vi "FTW-Request-Core-InterpretResponse.vi"(0 "Raw Response":T1, 5 "Expected Request Header":string, 11 "error in":errorcluster) -> (4 "InterpretedResponse":T1, 15 "error out":errorcluster)   [LabVIEW 2015]
doc: "Sends a response message back to the requesting client. This message is attempts to send unconditionally of incoming error. Take caution to wire a sanitized error into this function, because it will be repeated back onto the client. Said another way, an error generated while processing the request will be not only thrown on the request handler, but also on the client as well."
uses:
  core/type/FTW-Type-JSON.ctl
  error/FTW-ERR-ExceptionType.ctl
panel:
  # "Inputs"
  # "Outputs"
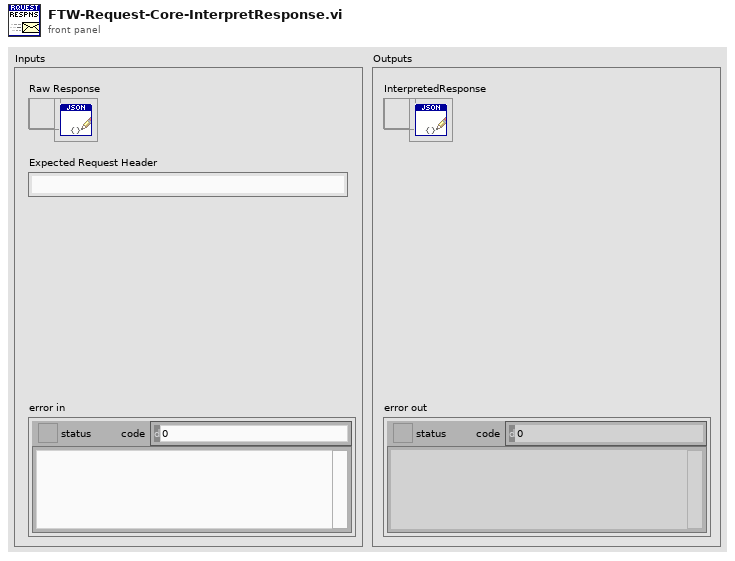
[diagram p1: front panel]
types:
  T1 = typedef "FTW-Type-JSON.ctl" = refnum<data-value>
  T2 = typedef "FTW-JSON-Type.ctl" = enum8{"Not Found", "Object", "Array", "String", "Number", "Boolean", "null"}
  T3 = typedef "FTW-ERR-ExceptionType.ctl" = enum16{"OK", "Info", "Warning", "Error"}
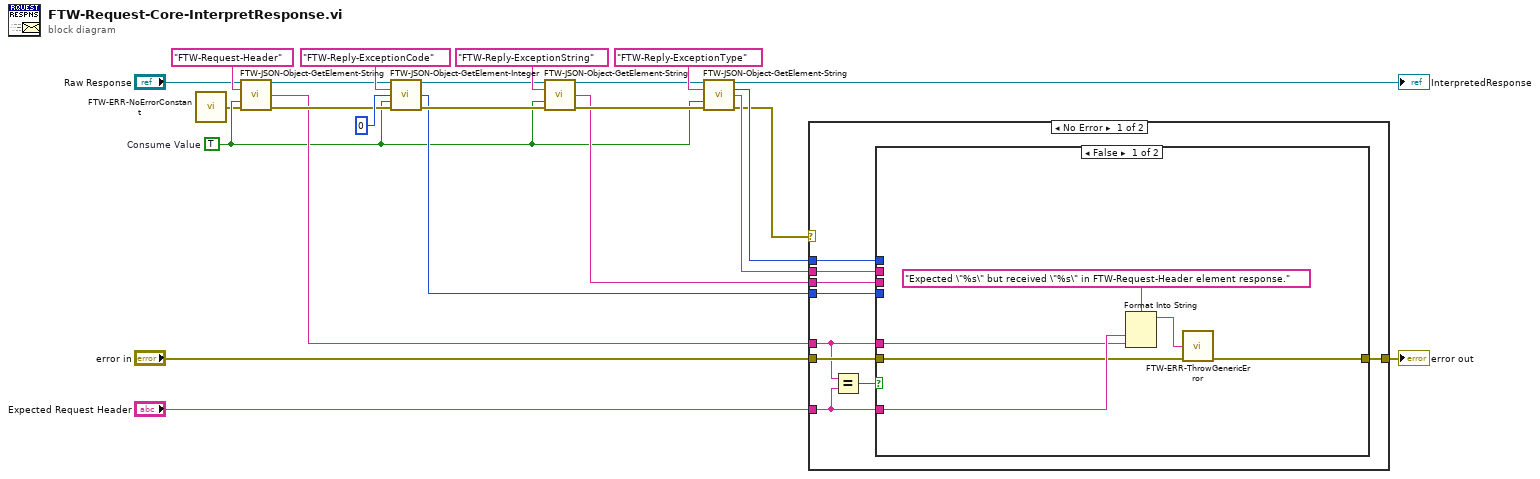
[diagram p0: block diagram]
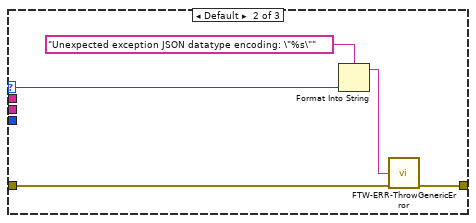
[diagram p3: hidden frame]
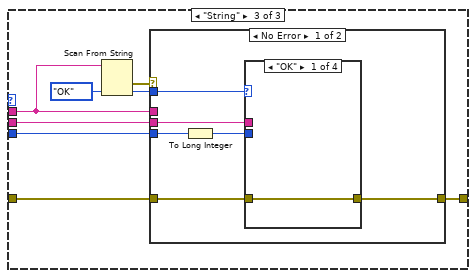
[diagram p4: hidden frame]
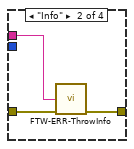
[diagram p5: hidden frame]
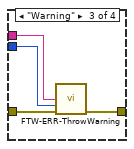
[diagram p6: hidden frame]
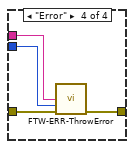
[diagram p7: hidden frame]
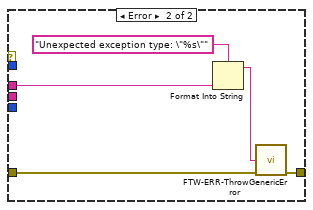
[diagram p8: hidden frame]
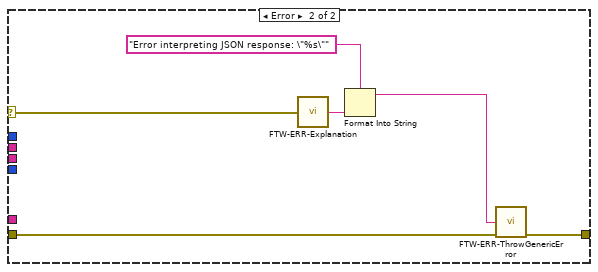
[diagram p9: hidden frame]
diagram:
  w5 = TRUE  # Consume Value
  n1 = call "FTW-ERR-NoErrorConstant.vi"() -> ("no error"=w3:errorcluster)
  n2 = call "FTW-JSON-Object-GetElement-String.vi"("JSON"="Raw Response", "Key"="FTW-Request-Header", "Consume Value"=w5, "error in"=w3) -> ("JSON out"=w8:T1, "Value"=w6:string, "error out"=w7:errorcluster)  [unwired: 8 in, 1 out]
  n3 = call "FTW-JSON-Object-GetElement-Integer.vi"("JSON"=w8, "Key"="FTW-Reply-ExceptionCode", "Default Value"=i64 0, "Consume Value"=w5, "error in"=w7) -> ("JSON out"=w18:T1, "Value"=w13:i64, "error out"=w17:errorcluster)  [unwired: 7 in, 1 out]
  n4 = call "FTW-JSON-Object-GetElement-String.vi"("JSON"=w18, "Key"="FTW-Reply-ExceptionString", "Consume Value"=w5, "error in"=w17) -> ("JSON out"=w15:T1, "Value"=w12:string, "error out"=w14:errorcluster)  [unwired: 8 in, 1 out]
  n5 = call "FTW-JSON-Object-GetElement-String.vi"("JSON"=w15, "Key"="FTW-Reply-ExceptionType", "Consume Value"=w5, "error in"=w14) -> ("JSON out"=→"InterpretedResponse":T1, "JSON Element Type"=w10:T2, "Value"=w11:string, "error out"=w2:errorcluster)  [unwired: 8 in]
  n6 = case shown="No Error" w2 {
    selector: w2 -> [_ w84]
    tunnel: [w30 w85] -> w23
    tunnel: "error in" -> [w31 w88]
    tunnel: w13 -> [w33 _]
    tunnel: w12 -> [w29 _]
    tunnel: w11 -> [w28 _]
    tunnel: w10 -> [w32 _]
    tunnel: w6 -> [w25 _]
    tunnel: "Expected Request Header" -> [w26 _]
    frame No Error {
      n7 = Equal?(x=w25, y=w26) -> (x = y?=w27:bool)
      n8 = case shown="False" w27 {
        tunnel: w33 -> [_ w45]
        tunnel: w32 -> [_ w44]
        tunnel: w31 -> [w35 w43]
        tunnel: [w34 w42] -> w30
        tunnel: w29 -> [_ w41]
        tunnel: w28 -> [_ w40]
        tunnel: w26 -> [w37 _]
        tunnel: w25 -> [w36 _]
        frame False {
          n9 = Format Into String(format string="Expected \"%s\" but received \"%s\" in FTW-Request-Header element response.", w37, w36) -> (resulting string=w39:string)  [unwired: 2 in, 1 out]
          n10 = call "FTW-ERR-ThrowGenericError.vi"("Error Message"=w39, "error in"=w35) -> ("error out"=w34:errorcluster)  [unwired: 13 in]
        }
        frame True {
          n11 = case shown="\"Not Found\", \"null\"" w44 {
            selector: w44 -> [_ w48 _]
            tunnel: w43 -> [w46 w51 w57]
            tunnel: [w46 w50 w56] -> w42
            tunnel: w40 -> [_ _ w55]
            tunnel: w41 -> [_ _ w53]
            tunnel: w45 -> [_ _ w52]
            frame "Not Found", "null" {
              # "No Exception"
            }
            frame Default {
              n12 = Format Into String(format string="Unexpected exception JSON datatype encoding: \"%s\"", w48) -> (resulting string=w47:string)  [unwired: 2 in, 1 out]
              n13 = call "FTW-ERR-ThrowGenericError.vi"("Error Message"=w47, "error in"=w51) -> ("error out"=w50:errorcluster)  [unwired: 13 in]
            }
            frame "String" {
              n14 = Scan From String(input string=w55, default 1=FTW-ERR-ExceptionType."OK" ("Exception")) -> (error out=w58:errorcluster, output 1=w54:T3)  [unwired: 3 in, 2 out]
              n15 = case shown="No Error" w58 {
                tunnel: w57 -> [w63 w82]
                tunnel: [w64 w81] -> w56
                tunnel: w55 -> [_ w78]
                tunnel: w54 -> [w65 _]
                tunnel: w52 -> [w61 _]
                tunnel: w53 -> [w62 _]
                frame No Error {
                  n16 = To Long Integer(number=w61) -> (32bit integer=w60:i32)
                  n17 = case shown="\"OK\"" w65 {
                    tunnel: [w66 w68 w72 w76] -> w64
                    tunnel: w63 -> [w66 w69 w73 w77]
                    tunnel: w62 -> [_ w67 w71 w75]
                    tunnel: w60 -> [_ _ w70 w74]
                    frame "OK" {
                    }
                    frame "Info" {
                      n18 = call "FTW-ERR-ThrowInfo.vi"("Informational Message"=w67, "error in"=w69) -> ("error out"=w68:errorcluster)  [unwired: 13 in]
                    }
                    frame "Warning" {
                      n19 = call "FTW-ERR-ThrowWarning.vi"("Warning Message"=w71, "Warning Code"=w70, "error in"=w73) -> ("error out"=w72:errorcluster)  [unwired: 12 in]
                    }
                    frame "Error" {
                      n20 = call "FTW-ERR-ThrowError.vi"("Error Message"=w75, "Error Code"=w74, "error in"=w77) -> ("error out"=w76:errorcluster)  [unwired: 12 in]
                    }
                  }
                }
                frame Error {
                  n21 = Format Into String(format string="Unexpected exception type: \"%s\"", w78) -> (resulting string=w79:string)  [unwired: 2 in, 1 out]
                  n22 = call "FTW-ERR-ThrowGenericError.vi"("Error Message"=w79, "error in"=w82) -> ("error out"=w81:errorcluster)  [unwired: 13 in]
                }
              }
            }
          }
        }
      }
    }
    frame Error {
      n23 = call "FTW-ERR-Explanation.vi"("error to check"=w84) -> ("Explanation"=w83:string)
      n24 = Format Into String(format string="Error interpreting JSON response: \"%s\"", w83) -> (resulting string=w86:string)  [unwired: 2 in, 1 out]
      n25 = call "FTW-ERR-ThrowGenericError.vi"("Error Message"=w86, "error in"=w88) -> ("error out"=w85:errorcluster)  [unwired: 13 in]
    }
  }
  "error out" <- w23
